vi "Standard Setup.vi"(8 "error in (no error)":errorcluster, 9 "Previous SET parameters":T1={"COOLER_POWER_STATUS"=0, "TEMP"=20, "EXPTIME"=1.0, "#FRAMES"=1, "#CUBES"=1}, 10 "Previous CCD Config":T5={"PREAMP"=enum."Gain 1", "READOUT_RATE"=enum."1 MHz", "EM_GAIN"=2, "VBIN"=1, "INITIAL_LINE"=1, "INITIAL_COLUMN"=1, "FINAL_LINE"=1024, "FINAL_COLUMN"=1024, "TRIGGER_MODE"=enum."Internal", "HBIN"=1, "SHUTTER_TTL"=enum."TTL Low", "SHUTTER_MODE"=enum."Close", "SHUTTER_OPENING_TIME"=50, "SHUTTER_CLOSING_TIME"=50, "VERTICAL_SHIFT_SPEED"=3, "READ_MODE"=enum."Image", "FRAME_TRANSFER"=TRUE, "VERTICAL_CLOCK_VOLTAGE"=enum."0", "ACQUISITION_MODE"=enum."Kinetics", "AD_CHANNEL"=0, "EM_MODE"=enum."Electron Multiplying"}, 11 "CCDCamera in":refnum<class "Simulated_CCD_Camera.lvclass">) -> (0 "error out":errorcluster, 3 "CCDCamera out":refnum<class "Simulated_CCD_Camera.lvclass">)   [LabVIEW 2018, in "Simulated_CCD_Camera.lvclass"]
uses:
  Simulated_CCD_Camera.lvclass
  <userlib>/atmcd32d.llb/Shutter_mode typedef.ctl
  <userlib>/atmcd32d.llb/ReadMode_mode typedef.ctl
  <userlib>/atmcd32d.llb/AcquisitionMode_mode typedef.ctl
  Simulated_CCD_Camera.lvclass/Simulated_CCD_Camera.ctl
  Interface/Interface.lvclass/Interface.ctl
  Interface/Interface.lvclass
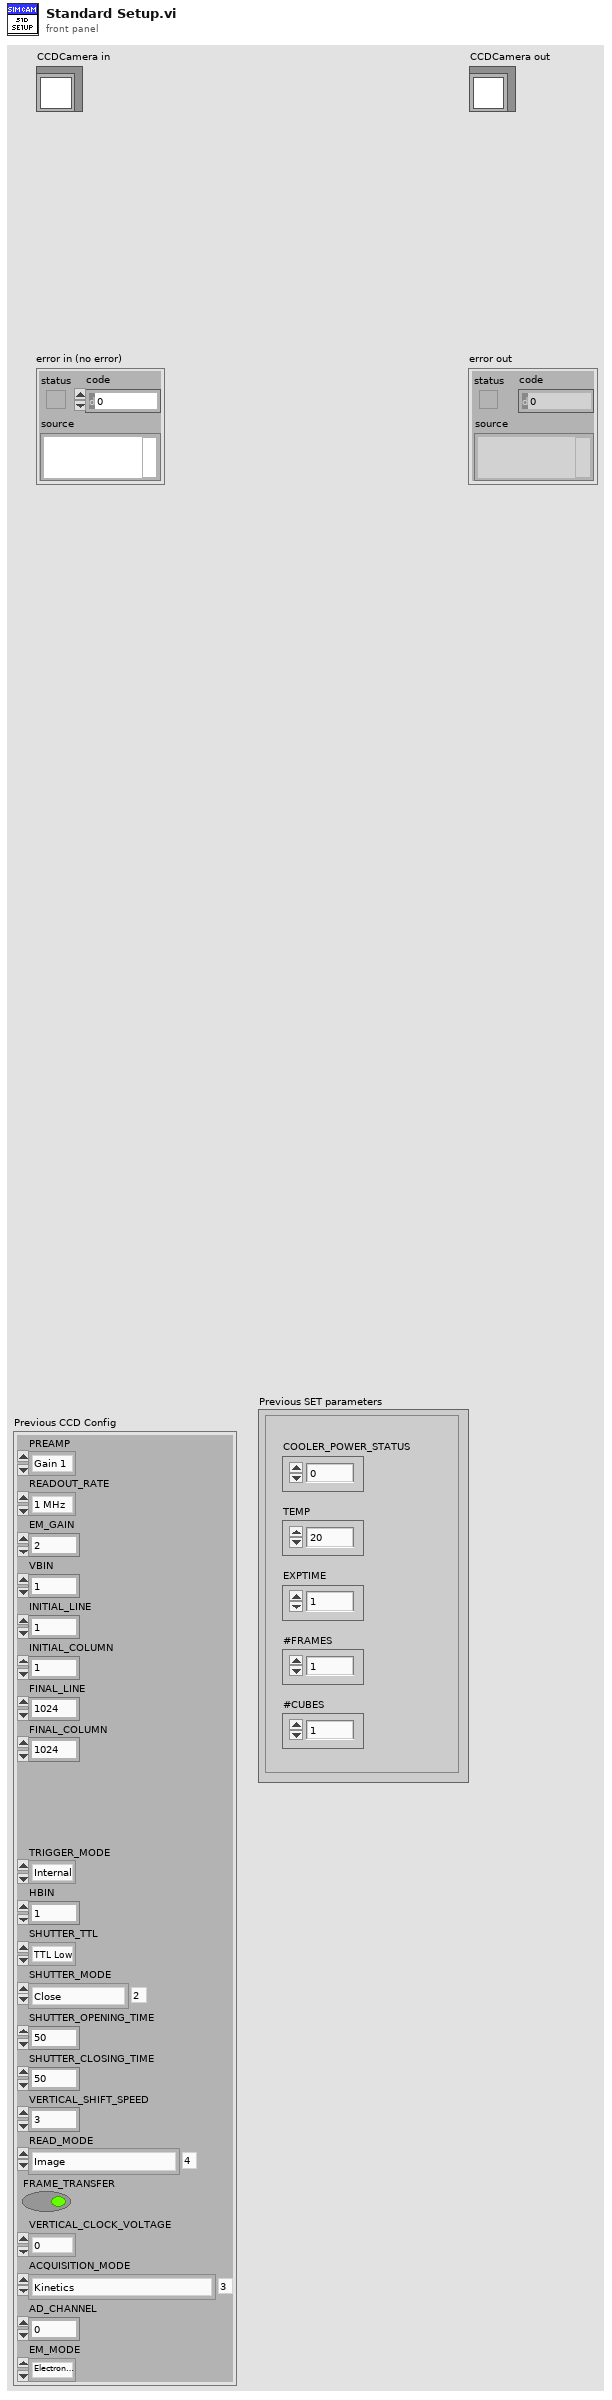
[diagram p1: front panel]
types:
  T1 = cluster{"COOLER_POWER_STATUS":u16, "TEMP":i32, "EXPTIME":dbl, "#FRAMES":u32, "#CUBES":u32}
  T2 = typedef "Shutter_mode typedef.ctl" = enum16{"Auto", "Open", "Close", "N/A (3)", "Open FVB Series", "Open Any Series"}
  T3 = typedef "ReadMode_mode typedef.ctl" = enum16{"Full Vertical Binning", "Multi-Track", "Random-Track", "Single-Track", "Image"}
  T4 = typedef "AcquisitionMode_mode typedef.ctl" = enum16{"Reserved (0)", "Single Scan", "Accumulate", "Kinetics", "Fast Kinetics", "Run Till Abort", "Reserved (6)", "Reserved (7)", "Reserved (8)", "Time Delayed Integration"}
  T5 = cluster{"PREAMP":enum16{"Gain 1", "Gain 2"}, "READOUT_RATE":enum16{"30 MHz", "20 MHz", "10 MHz", "1 MHz"}, "EM_GAIN":u16, "VBIN":u16, "INITIAL_LINE":u16, "INITIAL_COLUMN":u16, "FINAL_LINE":u16, "FINAL_COLUMN":u16, "TRIGGER_MODE":enum16{"Internal", "External", "N/A", "N/A_1", "N/A_2", "N/A_3", "External Start"}, "HBIN":u16, "SHUTTER_TTL":enum16{"TTL Low", "TTL High"}, "SHUTTER_MODE":T2, "SHUTTER_OPENING_TIME":u16, "SHUTTER_CLOSING_TIME":u16, "VERTICAL_SHIFT_SPEED":u16, "READ_MODE":T3, "FRAME_TRANSFER":bool, "VERTICAL_CLOCK_VOLTAGE":enum16{"0", "+1", "+2", "+3", "+4"}, "ACQUISITION_MODE":T4, "AD_CHANNEL":u16, "EM_MODE":enum16{"Electron Multiplying", "Conventional"}}
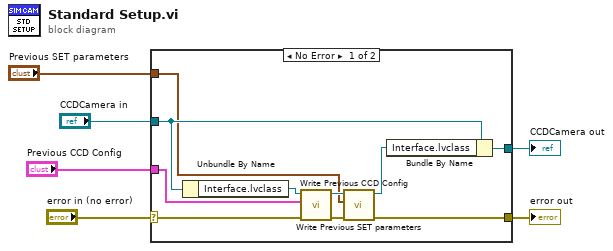
[diagram p0: block diagram]
diagram:
  n1 = case shown="No Error" "error in (no error)" {
    selector: "error in (no error)" -> [w13 w18]
    tunnel: [w9 w18] -> w4
    tunnel: [w15 w17] -> w3
    tunnel: "CCDCamera in" -> [w16 w17]
    tunnel: "Previous CCD Config" -> [w12 _]
    tunnel: "Previous SET parameters" -> [w7 _]
    frame No Error {
      n2 = Unbundle By Name(w16) -> ("Interface.lvclass"=w14:refnum<class "Interface.lvclass">)
      n3 = call "Write Previous CCD Config.vi"("error in (no error)"=w13, "Previous CCD Config"=w12, "Interface in"=w14) -> ("error out"=w10:errorcluster, "Interface out"=w11:refnum<class "Interface.lvclass">)  [unwired: 7 in]
      n4 = call "Write Previous SET parameters.vi"("error in (no error)"=w10, "Previous SET parameters"=w7, "Interface in"=w11) -> ("error out"=w9:errorcluster, "Interface out"=w8:refnum<class "Interface.lvclass">)  [unwired: 7 in]
      n5 = Bundle By Name(cluster=w16, "Interface.lvclass"=w8) -> (w15:refnum<class "Simulated_CCD_Camera.lvclass">)
    }
    frame Error {
    }
  }
  "error out" <- w4
  "CCDCamera out" <- w3
